vi "Read Periodic Delay Parameters.vi"(11 "Abstract Delay Line in":refnum<class "Abstract Delay Line.lvclass">) -> (2 "Periodic Delay Parameters":cluster{"Range (ps)":dbl, "Offset (ps)":dbl}, 3 "Abstract Delay Line out":refnum<class "Abstract Delay Line.lvclass">)   [LabVIEW 2016, in "Delay Line.lvlib" / "Abstract Delay Line.lvclass"]
uses:
  Abstract Delay Line.lvclass
  Abstract Delay Line.lvclass/Abstract Delay Line.ctl
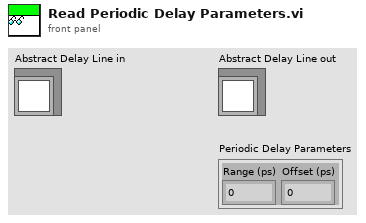
[diagram p1: front panel]
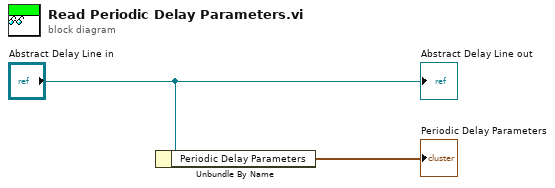
[diagram p0: block diagram]
diagram:
  n1 = Unbundle By Name("Abstract Delay Line in") -> ("Periodic Delay Parameters"=→"Periodic Delay Parameters":cluster{"Range (ps)":dbl, "Offset (ps)":dbl})
  "Abstract Delay Line out" <- "Abstract Delay Line in"
